vi "Get Attribute STRING.vi"(8 "error in":errorcluster, 10 "Attribute":string, 11 "Config from EXCEL in":refnum<class "Config from EXCEL.lvclass">) -> (0 "error out":errorcluster, 2 "Value":string, 3 "Config from EXCEL out":refnum<class "Config from EXCEL.lvclass">)   [LabVIEW 2025, in "Config from EXCEL.lvclass"]
uses:
  Config from EXCEL.lvclass
  Config from EXCEL.lvclass/Config from EXCEL.ctl
  Open-Xml-LabVIEW/Source/Open Xml.lvlib
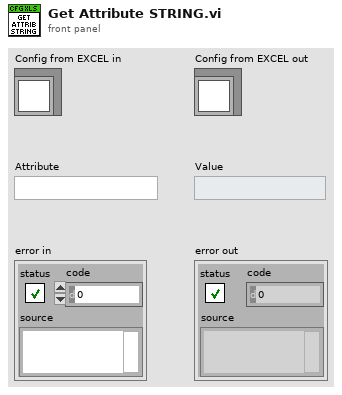
[diagram p1: front panel]
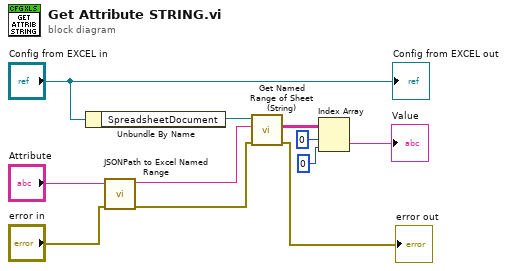
[diagram p0: block diagram]
diagram:
  n1 = Unbundle By Name("Config from EXCEL in") -> ("SpreadsheetDocument"=w8:refnum<k24>)
  n2 = call "JSONPath to Excel Named Range.vi"("error in"="error in", "JSONPath"="Attribute") -> ("error out"=w2:errorcluster, "Named Range"=w7:string)  [unwired: 8 in]
  n3 = call "Get Named Range of Sheet (String).vi"("error in"=w2, "Named Range Identifier"=w7, "SpreadsheetDocument"=w8) -> ("error out"=→"error out":errorcluster, "Cells"=w6:string[][])  [unwired: 6 in, 1 out]
  n4 = Index Array(array=w6, index (row)=0, index (col)=0) -> (element=→"Value":string)
  "Config from EXCEL out" <- "Config from EXCEL in"
